vi "Log Event.vi"(8 "Clear Log":bool, 9 "Message":string, 10 "Log Level":T1, 11 "Read":bool) -> (2 "All Events":string[](array[string]))   [LabVIEW 2021]
uses:
  Log Level.ctl
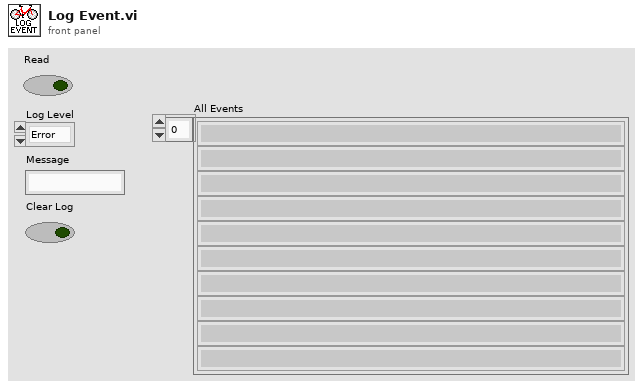
[diagram p1: front panel]
types:
  T1 = typedef "Log Level.ctl" = enum16{"Error", "Warning", "Info"}
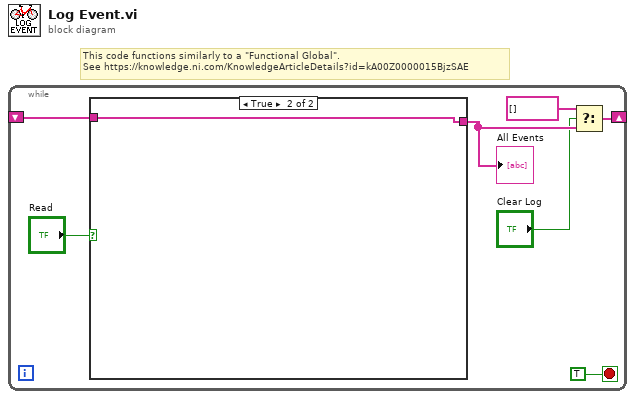
[diagram p0: block diagram]
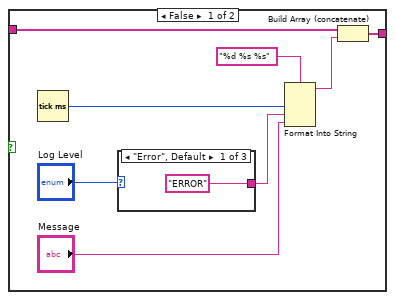
[diagram p2: hidden frame]
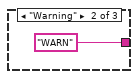
[diagram p3: hidden frame]
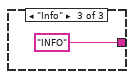
[diagram p4: hidden frame]
diagram:
  # "This code functions similarly to a \"Functional Global\".\nSee https://knowledge.ni.com/KnowledgeArticleDetails?id=kA00Z0000015BjzSAE"
  n1 = while {
    shift-right: [w5] -> _
    shift-left: _ -> [w6]
    stop <- TRUE stop-if-true
    n2 = case shown="True" "Read" {
      tunnel: w6 -> [w15 w19]
      tunnel: [w8 w19] -> w4
      frame False {
        n3 = Tick Count (ms)() -> (millisecond timer value=w13:u32)
        n4 = case shown="\"Error\", Default" "Log Level" {
          tunnel: ["ERROR" "WARN" "INFO"] -> w10
          frame "Error", Default {
          }
          frame "Warning" {
          }
          frame "Info" {
          }
        }
        n5 = Format Into String(format string="%d %s %s", w13, w10, "Message") -> (resulting string=w9:string)  [unwired: 2 in, 1 out]
        n6 = Build Array (concatenate)(w15, w9) -> (w8:string[])
      }
      frame True {
      }
    }
    "All Events" <- w4
    n7 = Select(t=string[] [], s="Clear Log", f=w4) -> (s? t:f=w5:string[])
  }
